vi "BBox.vi"() -> ()   [LabVIEW 2021]
panel:
  in  "Python version":u16(ring)=2 items=["3.6", "3.7", "3.8", "3.9"]
  in  "Gain":sgl min=-20 max=30 step=0.5 format="%2.1g"
  out "Beam result":bool
  out "AAKit result":bool
  out "Freq result":bool
  out "T/R result":bool
  out "init result":bool
  out "Final state":bool
  in  "TX/RX switch":bool
  in  "Frequency(GHz)":sgl=28.0 min=26.5 max=29.5 step=0.5 format="%#_3f"
  in  "error in (no error)":errorcluster
  in  "Please assign module path (TLKCore_vx.x.x_xxx/main.py)":path=path "C:/TLKCore/main.py"
  in  "Phi":i16 min=0 max=360 step=1 format="%3d"
  in  "Theta":i16 min=0 max=60 step=1 format="%2d"
  out "DR range":sgl[](array[numeric]) caption="Dynamic Range (dB)"
  in  "Please input AAKit Name":string="AAKIT_TMYTEK-4x4_ONE_28_IDEAL"
  out "Current AAKit List":string[](array[string])
  in  "Please assign SN":string="D2230E013-28"
  out "Scanned List (SN,IP,dev_type)":string[](array[string])
  out "Exception message":T1
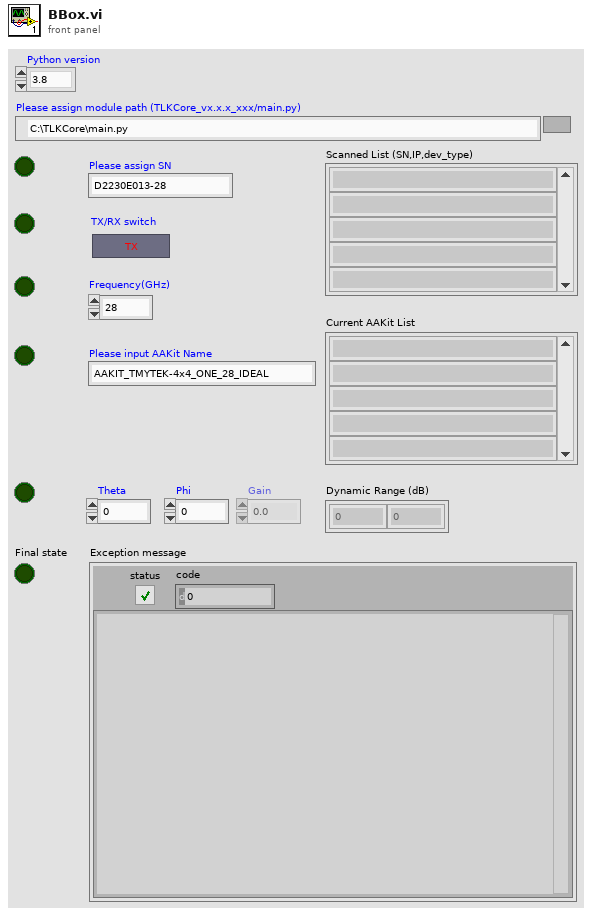
[diagram p1: front panel]
types:
  T1 = cluster{"status":bool, "code":i32, "Exception message":string}
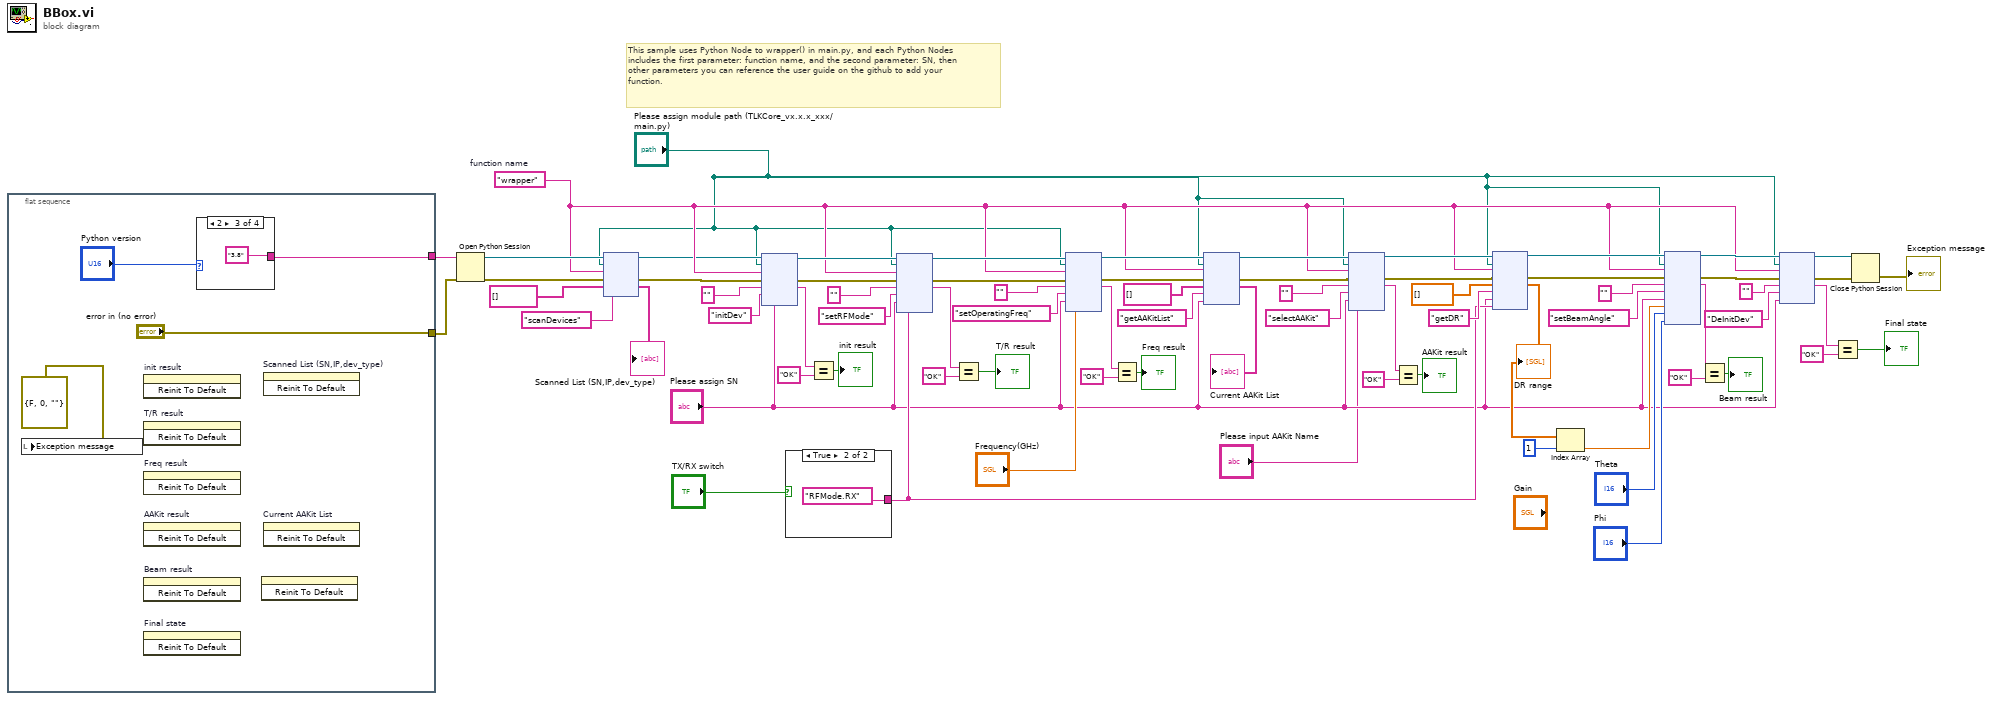
[diagram p0: block diagram]
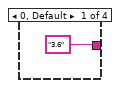
[diagram p2: hidden frame]
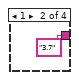
[diagram p3: hidden frame]
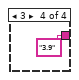
[diagram p4: hidden frame]
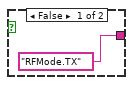
[diagram p5: hidden frame]
diagram:
  w36 = "wrapper"  # function name
  # "This sample uses Python Node to wrapper() in main.py, and each Python Nodes includes the first parameter: function name, and the second parameter: SN, then other parameters you can reference the user guide on the github to add your function."
  n1 = flat-sequence {
    tunnel: ["error in (no error)"] -> w27
    tunnel: [w75] -> w1
    frame #0 {
      n2 = local write "Exception message"(errorcluster {"status"=FALSE, "code"=0, "source"=""} ("Exception message")) -> ()
      n3 = invoke on="init result" class="Bool (strict)" method="Reinit To Default"() -> ()  [unwired: 3 in, 3 out]
      n4 = invoke on="T/R result" class="Bool (strict)" method="Reinit To Default"() -> ()  [unwired: 3 in, 3 out]
      n5 = invoke on="Freq result" class="Bool (strict)" method="Reinit To Default"() -> ()  [unwired: 3 in, 3 out]
      n6 = invoke on="AAKit result" class="Bool (strict)" method="Reinit To Default"() -> ()  [unwired: 3 in, 3 out]
      n7 = invoke on="Beam result" class="Bool (strict)" method="Reinit To Default"() -> ()  [unwired: 3 in, 3 out]
      n8 = invoke on="Final state" class="Bool (strict)" method="Reinit To Default"() -> ()  [unwired: 3 in, 3 out]
      n9 = case shown="2" "Python version" {
        tunnel: ["3.6" ("python version") "3.7" ("python version") "3.8" ("python version") "3.9" ("python version")] -> w75
        frame 0, Default {
        }
        frame 1 {
        }
        frame 2 {
        }
        frame 3 {
        }
      }
      n10 = invoke on="DR range" class="Arr (strict)" method="Reinit To Default"() -> ()  [unwired: 3 in, 3 out]
      n11 = invoke on="Scanned List (SN,IP,dev_type)" class="Arr (strict)" method="Reinit To Default"() -> ()  [unwired: 3 in, 3 out]
      n12 = invoke on="Current AAKit List" class="Arr (strict)" method="Reinit To Default"() -> ()  [unwired: 3 in, 3 out]
    }
  }
  n13 = Open Python Session(python version=w1, 3:w27) -> (session out=w73:refnum<k35>, error out=w72:errorcluster)  [unwired: 1 in]
  n14 = node ("Python Node")(w73, "Please assign module path (TLKCore_vx.x.x_xxx/main.py)", w36, w72, string[] [], "scanDevices") -> (w29:refnum<k35>, w71:errorcluster, →"Scanned List (SN,IP,dev_type)":string[])  [unwired: 1 in, 2 out]
  n15 = node(w29, "Please assign module path (TLKCore_vx.x.x_xxx/main.py)", w36, w71, "", "initDev", "Please assign SN") -> (w62:refnum<k35>, w63:errorcluster, w14:string)  [unwired: 2 in, 2 out]
  n16 = case shown="True" "TX/RX switch" {
    tunnel: ["RFMode.TX" ("RF Mode string") "RFMode.RX" ("RF Mode string")] -> w24
    frame False {
    }
    frame True {
    }
  }
  n17 = Equal?(x=w14, y="OK") -> (x = y?=→"init result":bool)
  n18 = node(w62, "Please assign module path (TLKCore_vx.x.x_xxx/main.py)", w36, w63, "", "setRFMode", "Please assign SN", w24) -> (w55:refnum<k35>, w54:errorcluster, w12:string)  [unwired: 3 in, 2 out]
  n19 = Equal?(x=w12, y="OK") -> (x = y?=→"T/R result":bool)
  n20 = node(w55, "Please assign module path (TLKCore_vx.x.x_xxx/main.py)", w36, w54, "", "setOperatingFreq", "Please assign SN", "Frequency(GHz)") -> (w49:refnum<k35>, w48:errorcluster, w9:string)  [unwired: 3 in, 2 out]
  n21 = Equal?(x=w9, y="OK") -> (x = y?=→"Freq result":bool)
  n22 = node(w49, "Please assign module path (TLKCore_vx.x.x_xxx/main.py)", w36, w48, string[] [], "getAAKitList", "Please assign SN") -> (w46:refnum<k35>, w45:errorcluster, →"Current AAKit List":string[])  [unwired: 2 in, 2 out]
  n23 = node(w46, "Please assign module path (TLKCore_vx.x.x_xxx/main.py)", w36, w45, "", "selectAAKit", "Please assign SN", "Please input AAKit Name") -> (w41:refnum<k35>, w42:errorcluster, w6:string)  [unwired: 3 in, 2 out]
  n24 = Equal?(x=w6, y="OK") -> (x = y?=→"AAKit result":bool)
  n25 = node(w41, "Please assign module path (TLKCore_vx.x.x_xxx/main.py)", w36, w42, sgl[] [], "getDR", "Please assign SN", w24) -> (w40:refnum<k35>, w39:errorcluster, w34:sgl[])  [unwired: 3 in, 2 out]
  "DR range" <- w34
  n26 = Index Array(array=w34, index=1) -> (element=w32:sgl)
  n27 = node(w40, "Please assign module path (TLKCore_vx.x.x_xxx/main.py)", w36, w39, "", "setBeamAngle", "Please assign SN", w32, "Theta", "Phi") -> (w37:refnum<k35>, w38:errorcluster, w3:string)  [unwired: 5 in, 2 out]
  n28 = Equal?(x=w3, y="OK") -> (x = y?=→"Beam result":bool)
  n29 = node(w37, "Please assign module path (TLKCore_vx.x.x_xxx/main.py)", w36, w38, "", "DeInitDev", "Please assign SN") -> (w59:refnum<k35>, w58:errorcluster, w19:string)  [unwired: 2 in, 2 out]
  n30 = Equal?(x=w19, y="OK") -> (x = y?=→"Final state":bool)
  n31 = Close Python Session(session in=w59, error in=w58) -> (11:→"Exception message":errorcluster)
